vi "DLPIO20_Init.vi"(11 "VISA resource name":refnum<visa-resource-name>) -> (0 "error out":errorcluster, 2 "DLP FOUND":bool, 3 "VISA resource name out":refnum<visa-resource-name>)   [LabVIEW 2016, in "DLPIO20_PackedLibrary.lvlib"]
uses:
  DLPIO20_PackedLibrary.lvlib
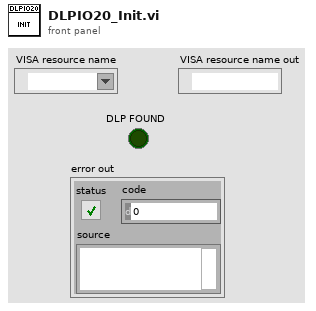
[diagram p1: front panel]
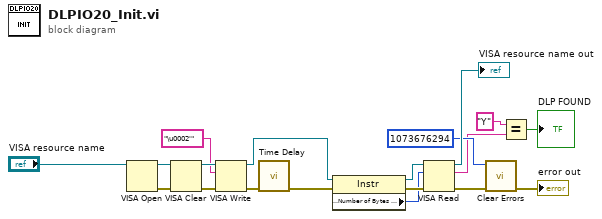
[diagram p0: block diagram]
diagram:
  n1 = VISA Open(VISA resource name="VISA resource name") -> (VISA resource name=w18:refnum<visa-resource-name>, error out=w17:errorcluster)  [unwired: 4 in]
  n2 = VISA Clear(VISA resource name=w18, error in (no error)=w17) -> (VISA resource name out=w15:refnum<visa-resource-name>, error out=w16:errorcluster)
  n3 = VISA Write(VISA resource name=w15, write buffer="\u0002'", error in (no error)=w16) -> (VISA resource name out=w8:refnum<visa-resource-name>, error out=w13:errorcluster)  [unwired: 1 out]
  n4 = call "Time Delay"("error in (no error)"=w13) -> ("error out"=w7:errorcluster)  [unwired: 10 in]
  n5 = property class="Instr"(reference=w8, error in=w7) -> (reference out=w11:refnum<visa-resource-name>, error out=w10:errorcluster, "Serial Settings:Number of Bytes at Serial Port"=w9:u32)
  n6 = VISA Read(VISA resource name=w11, byte count=w9, error in (no error)=w10) -> (VISA resource name out=→"VISA resource name out":refnum<visa-resource-name>, read buffer=w3:string, error out=w5:errorcluster)  [unwired: 1 out]
  n7 = call <vilib>:"Clear Errors.vi"("error in (no error)"=w5, "specific error code to clear (0: all)"=1073676294) -> ("error out"=→"error out":errorcluster)  [unwired: 4 in, 1 out]
  n8 = Equal?(x="Y", y=w3) -> (x = y?=→"DLP FOUND":bool)
